vi "sv_Init Relative Response (Octave).vi"(0 "octave spectrum":T5, 5 "weighting filter":u16, 9 "octave info":T1={"standard"=enum."ANSI S1.11", "bandwidth"=enum."1 octave", "low band"=0, "high band"=0, "weighting filter"=0, "dB reference"=0.0, "dB On"=FALSE, "unit label"="", "channel name"="", "description"="", "engineering units"=1, "custom label"="", "spectrum type"=enum."magnitude", "spectral density"=FALSE, "filters settled"=FALSE} {"engineering units" items=["custom..."=0, "V"=1, "A"=21, "C"=30, "pC"=31, "s"=32, "-"=29, "Pa"=2, "N"=20, "g"=3, "m/s^2"=4, "m/s"=5, "m"=6, "mm/s"=12, "mm"=13, "micron/s"=14, "micron"=15, "in/s^2"=7, "in/s"=8, "in"=9, "mil/s"=10, "mil"=11, "rad/s^2"=16, "rad/s"=17, "rad"=18, "deg/s^2"=26, "deg/s"=27, "deg"=28, "RPM"=22, "cycle/s^2"=23, "Hz"=24, "cycle"=25, "strain"=19]; "dB reference" format="%.2e"; "weighting filter" items=["Linear", "A-weighting", "B-weighting", "C-weighting", "ITU-R 468-4", "Dolby", "CCITT", "C-message", "Wb", "Wc", "Wd", "We", "Wf", "Wh", "Wj", "Wk", "Wm", "AES17 20 kHz lowpass", "AES17 40 kHz lowpass", "AES17 20 kHz highpass", "AES17 40 kHz highpass"]}, 11 "error in (no error)":errorcluster, 12 "reset":bool) -> (4 "dup octave spectrum":T5, 6 "dup weighting filter":u16, 8 "relative response":dbl[](array[numeric]), 10 "dup octave info":T1={"standard"=enum."ANSI S1.11", "bandwidth"=enum."1 octave", "low band"=0, "high band"=0, "weighting filter"=0, "dB reference"=0.0, "dB On"=FALSE, "unit label"="", "channel name"="", "description"="", "engineering units"=1, "custom label"="", "spectrum type"=enum."magnitude", "spectral density"=FALSE, "filters settled"=FALSE} {"engineering units" items=["custom..."=0, "V"=1, "A"=21, "C"=30, "pC"=31, "s"=32, "-"=29, "Pa"=2, "N"=20, "g"=3, "m/s^2"=4, "m/s"=5, "m"=6, "mm/s"=12, "mm"=13, "micron/s"=14, "micron"=15, "in/s^2"=7, "in/s"=8, "in"=9, "mil/s"=10, "mil"=11, "rad/s^2"=16, "rad/s"=17, "rad"=18, "deg/s^2"=26, "deg/s"=27, "deg"=28, "RPM"=22, "cycle/s^2"=23, "Hz"=24, "cycle"=25, "strain"=19]; "dB reference" format="%.2e"; "weighting filter" items=["Linear", "A-weighting", "B-weighting", "C-weighting", "ITU-R 468-4", "Dolby", "CCITT", "C-message", "Wb", "Wc", "Wd", "We", "Wf", "Wh", "Wj", "Wk", "Wm", "AES17 20 kHz lowpass", "AES17 40 kHz lowpass", "AES17 20 kHz highpass", "AES17 40 kHz highpass"]}, 15 "error out":errorcluster)   [LabVIEW 2017]
uses:
  <vilib>/addons/_NISVFA/_Shared subVIs/Controls/svc_Octave Info.ctl
  <vilib>/addons/_NISVFA/_Shared subVIs/Controls/svc_Octave Standard.ctl
  <vilib>/addons/_NISVFA/_Shared subVIs/Controls/svc_Weighting Filter Text Ring.ctl
  <vilib>/addons/_NISVFA/_Shared subVIs/Controls/svc_Engineering Units Text Ring.ctl
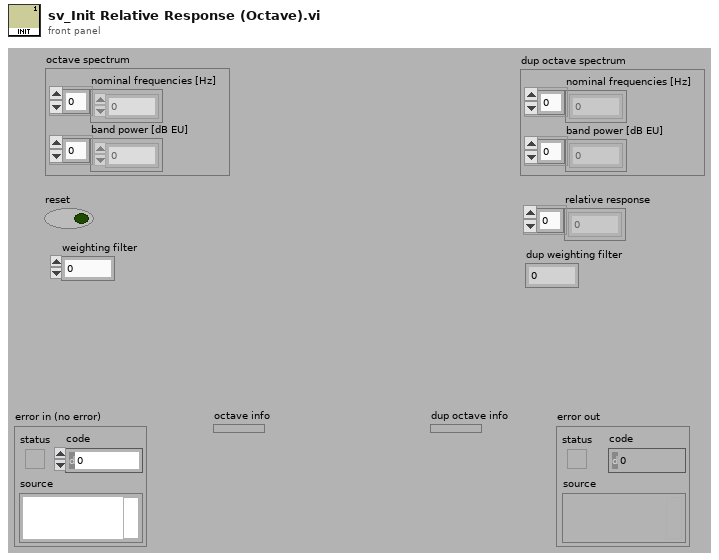
[diagram p1: front panel]
types:
  T1 = typedef "svc_Octave Info.ctl" = cluster{"standard":T2, "bandwidth":enum16{"1 octave", "1/3 octave", "1/6 octave", "1/12 octave", "1/24 octave"}, "low band":i32, "high band":i32, "weighting filter":T3, "dB reference":dbl, "dB On":bool, "unit label":string, "channel name":string, "description":string, "engineering units":T4, "custom label":string, "spectrum type":enum16{"power", "magnitude"}, "spectral density":bool, "filters settled":bool}
  T2 = typedef "svc_Octave Standard.ctl" = enum16{"ANSI S1.11", "IEC 61260"}
  T3 = typedef "svc_Weighting Filter Text Ring.ctl" = u16
  T4 = typedef "svc_Engineering Units Text Ring.ctl" = u16
  T5 = cluster{"nominal frequencies [Hz]":dbl[], "band power [dB EU]":dbl[]}
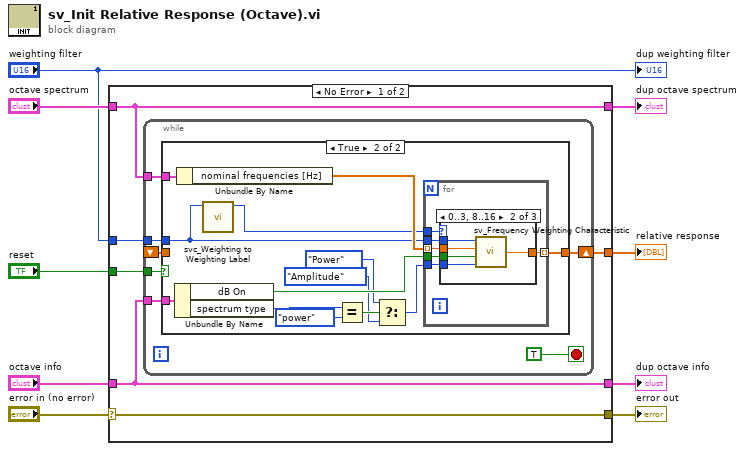
[diagram p0: block diagram]
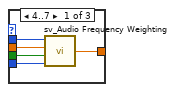
[diagram p3: hidden frame]
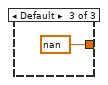
[diagram p4: hidden frame]
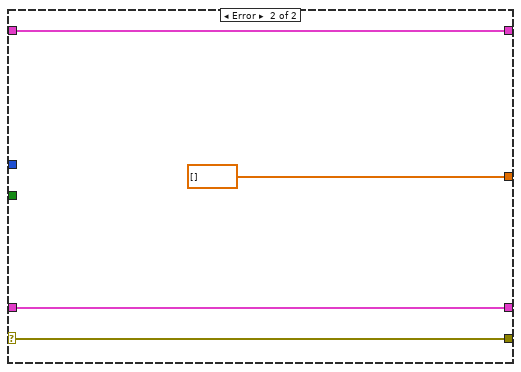
[diagram p5: hidden frame]
diagram:
  n1 = case shown="No Error" "error in (no error)" {
    selector: "error in (no error)" -> [w11 w54]
    tunnel: [w15 dbl[] []] -> w9
    tunnel: "octave spectrum" -> [w13 w57]
    tunnel: "octave info" -> [w12 w56]
    tunnel: "weighting filter" -> [w14 _]
    tunnel: [w13 w57] -> w6
    tunnel: [w12 w56] -> w5
    tunnel: [w11 w54] -> w3
    tunnel: "reset" -> [w10 _]
    frame No Error {
      n2 = while {
        tunnel: w14 -> [w21]
        tunnel: w13 -> [w20]
        tunnel: w12 -> [w19]
        tunnel: w10 -> [w18]
        shift-right: [w22] -> w15
        shift-left: _ -> [w16]
        stop <- TRUE stop-if-true
        n3 = case shown="True" w18 {
          tunnel: [w23 w36] -> w22
          tunnel: w21 -> [_ w33]
          tunnel: w20 -> [_ w31]
          tunnel: w19 -> [_ w30]
          tunnel: w16 -> [w23 _]
          frame False {
          }
          frame True {
            n4 = Unbundle By Name(w30) -> ("dB On"=w34:bool, "spectrum type"=w29:enum16{"power", "magnitude"})
            n5 = Unbundle By Name(w31) -> ("nominal frequencies [Hz]"=w35:dbl[])
            n6 = call <vilib>:"svc_Weighting to Weighting Label.vi"("weighting filter"=w33) -> ("weighting enum"=w32:T3)  [unwired: 9 in, 1 out]
            n7 = Equal?(x=w29, y=enum16{"power", "magnitude"}."power") -> (x = y?=w27:bool)
            n8 = Select(t=enum16{"Power", "Amplitude"}."Power" ("spectrum type"), s=w27, f=enum16{"Power", "Amplitude"}."Amplitude") -> (s? t:f=w24:enum16{"Power", "Amplitude"})
            n9 = for {
              tunnel: w33 -> [w42]
              tunnel: w34 -> [w40]
              tunnel: w35 -> [w41] mode=indexing
              tunnel: [w38] -> w36 mode=indexing
              tunnel: w24 -> [w39]
              tunnel: w32 -> [w37]
              n10 = case shown="0..3, 8..16" w37 {
                tunnel: [w43 w48 nan ("relative response level")] -> w38
                tunnel: w41 -> [w46 w52 _]
                tunnel: w42 -> [w47 w51 _]
                tunnel: w39 -> [w44 w50 _]
                tunnel: w40 -> [w45 w49 _]
                frame 4..7 {
                  n11 = call <vilib>:"sv_Audio Frequency Weighting.vi"("spectrum type"=w44, "dB On (T)"=w45, "frequency [Hz]"=w46, "weighting filter"=w47) -> ("relative response level"=w43:dbl)
                }
                frame 0..3, 8..16 {
                  n12 = call <vilib>:"sv_Frequency Weighting Characteristic.vi"("spectrum type"=w50, "dB On (T)"=w49, "frequency [Hz]"=w52, "weighting filter"=w51) -> ("relative response level"=w48:dbl)
                }
                frame Default {
                }
              }
            }
          }
        }
      }
    }
    frame Error {
    }
  }
  "relative response" <- w9
  "dup octave spectrum" <- w6
  "dup octave info" <- w5
  "error out" <- w3
  "dup weighting filter" <- "weighting filter"
